vi "Assert Global.vi"(10 "Set (F)":bool, 11 "Assert in":refnum<class "Assert.lvclass">) -> (1 "Is Set?":bool, 2 "Succeeded?":bool, 3 "Assert out":refnum<class "Assert.lvclass">)   [LabVIEW 2009]
uses:
  Assert/Assert.lvclass
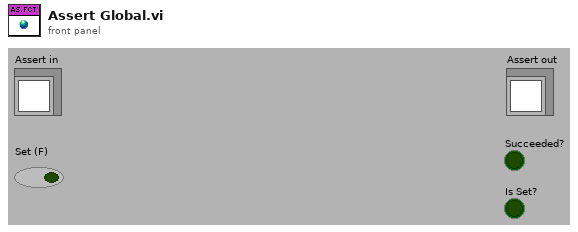
[diagram p1: front panel]
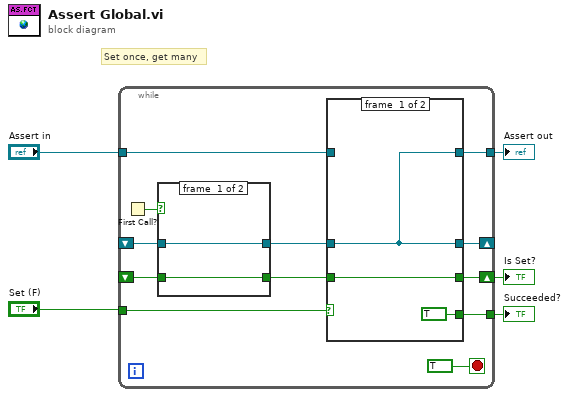
[diagram p0: block diagram]
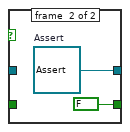
[diagram p2: hidden frame]
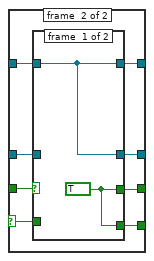
[diagram p3: hidden frame]
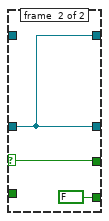
[diagram p4: hidden frame]
diagram:
  # "Set once, get many"
  n1 = while {
    tunnel: "Set (F)" -> [w16]
    tunnel: "Assert in" -> [w13]
    shift-right: [w11] -> _
    shift-left: _ -> [w14]
    tunnel: [w10] -> w3
    shift-right: [w8] -> w5
    shift-left: _ -> [w9]
    tunnel: [w6] -> w4
    stop <- TRUE stop-if-true
    n2 = First Call?() -> (First Call?: T/F=w15:bool)
    n3 = case shown="True" w15 {
      tunnel: w14 -> [w19 _]
      tunnel: [w19 w20] -> w12
      tunnel: w9 -> [w18 _]
      tunnel: [w18 FALSE] -> w7
      frame #0 {
      }
      frame #1 {
        w20 = refnum<class "Assert.lvclass"> refnum  # Assert
      }
    }
    n4 = case shown="True" w16 {
      selector: w16 -> [_ w26]
      tunnel: w13 -> [_ w32]
      tunnel: w12 -> [w24 w29]
      tunnel: [w24 w28] -> w11
      tunnel: [w24 w30] -> w10
      tunnel: [w23 w27] -> w8
      tunnel: w7 -> [w23 w31]
      tunnel: [TRUE w25] -> w6
      frame #0 {
      }
      frame #1 {
        n5 = case shown="False" w31 {
          selector: w31 -> [_ w36]
          tunnel: w32 -> [w34 _]
          tunnel: [w34 w37] -> w30
          tunnel: w29 -> [_ w37]
          tunnel: [w34 w37] -> w28
          tunnel: [w33 w36] -> w27
          tunnel: w26 -> [_ _]
          tunnel: [w33 FALSE] -> w25
          frame #0 {
            w33 = TRUE
          }
          frame #1 {
          }
        }
      }
    }
  }
  "Assert out" <- w3
  "Is Set?" <- w5
  "Succeeded?" <- w4
